vi "Base64_Encoding.vi"(0 "normal string":string) -> (2 "base64 string":string)   [LabVIEW 2020, in "DP_WebView.lvclass"]
doc: "Encodes a string to base64 format."
uses:
  DP_WebView.lvclass
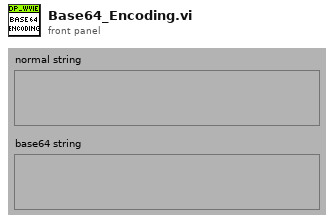
[diagram p1: front panel]
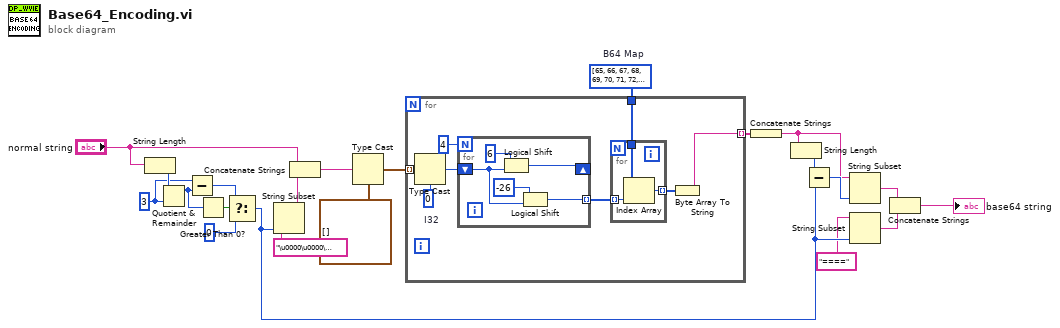
[diagram p0: block diagram]
diagram:
  w10 = u8[] [65, 66, 67, 68, 69, 70, 71, 72, 73, 74, 75, 76, 77, 78, 79, 80, 81, 82, 83, 84, 85, 86, 87, 88, 89, 90, 97, 98, 99, 100, 101, 102, 103, 104, 105, 106, 107, 108, 109, 110, 111, 112, 113, 114, 115, 116, 117, 118, 119, 120, 121, 122, 48, 49, 50, 51, 52, 53, 54, 55, 56, 57, 43, 47]  # B64 Map
  w16 = 3 ("y")
  n1 = String Length(string="normal string") -> (length=w17:i32)
  n2 = Quotient & Remainder(x=w17, y=w16) -> (x-y*floor(x/y)=w15:i32)  [unwired: 1 out]
  n3 = Subtract(x=w16, y=w15) -> (x-y=w12:i32)
  n4 = Greater Than 0?(x=w15) -> (x > 0?=w14:bool)
  n5 = Select(t=w12, s=w14, f=0 ("y")) -> (s? t:f=w7:i32)
  n6 = String Subset(string="\u0000\u0000\u0000\u0000", length (rest)=w7) -> (substring=w21:string)  [unwired: 1 out]
  n7 = Concatenate Strings("normal string", w21) -> (w19:string)
  n8 = Type Cast(type=cluster{"u8":u8, "u8":u8, "u8":u8}[] [], x=w19) -> (*(type *) &x=w11:cluster{"u8":u8, "u8":u8, "u8":u8}[])
  n9 = for {
    tunnel: w11 -> [w30] mode=indexing
    tunnel: w10 -> [w25]
    tunnel: [w23] -> w2 mode=indexing
    w29 = 0  # I32
    n10 = Type Cast(type=w29, x=w30) -> (*(type *) &x=w28:i32)
    n11 = for {
      N: 4 -> [_]
      shift-right: [w38] -> _
      shift-left: w28 -> [w35]
      tunnel: [w34] -> w26 mode=indexing
      n12 = Logical Shift(y=6, x=w35) -> (x << y=w38:i32)
      n13 = Logical Shift(y=-26, x=w35) -> (x << y=w34:i32)
    }
    n14 = for {
      tunnel: w26 -> [w33] mode=indexing
      tunnel: w25 -> [w32]
      tunnel: [w31] -> w24 mode=indexing
      n15 = Index Array(array=w32, index=w33) -> (element=w31:u8)
    }
    n16 = Byte Array To String(unsigned byte array=w24) -> (string=w23:string)
  }
  n17 = Concatenate Strings(w2) -> (w1:string)
  n18 = String Length(string=w1) -> (length=w9:i32)
  n19 = Subtract(x=w9, y=w7) -> (x-y=w8:i32)
  n20 = String Subset(string=w1, length (rest)=w8) -> (substring=w5:string)  [unwired: 1 out]
  n21 = String Subset(string="====", length (rest)=w7) -> (substring=w4:string)  [unwired: 1 out]
  n22 = Concatenate Strings(w5, w4) -> (→"base64 string":string)
